vi "Get DQMH Main VI QD.vi"(8 "error in (no error)":errorcluster, 11 "Library Ref in":refnum<vi>) -> (0 "error out":errorcluster, 2 "Main VI Ref":refnum<vi>, 3 "Library Ref out":refnum<vi>)   [LabVIEW 2017]
doc: "Returns the Main VI of the DQMH Module of the selected SubVI."
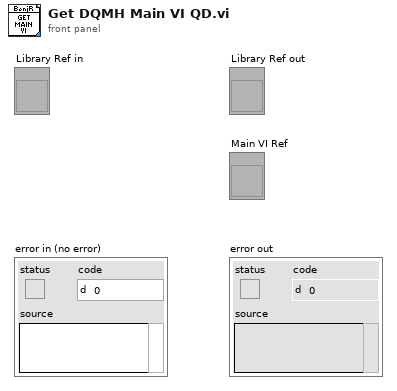
[diagram p1: front panel]
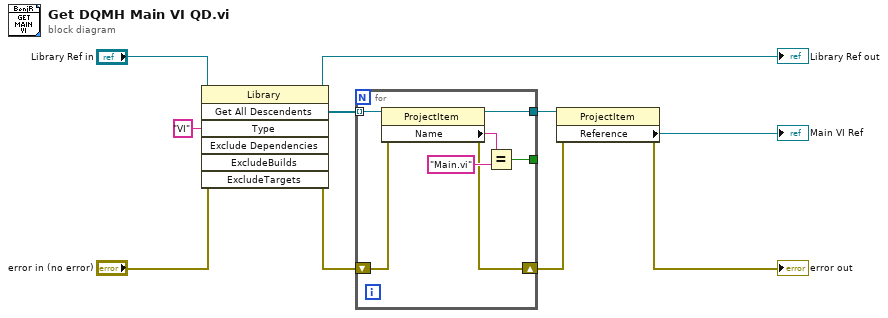
[diagram p0: block diagram]
diagram:
  n1 = invoke class="Library" method="Get All Descendents"(reference="Library Ref in", error in="error in (no error)", "Type"="VI") -> (reference out=→"Library Ref out":refnum<vi>, error out=w6:errorcluster, "All Descendents"=w3:refnum<vi>[])  [unwired: 4 in, 4 out]
  n2 = for {
    tunnel: w3 -> [w17] mode=indexing
    tunnel: [w14] -> _
    tunnel: [w13] -> w4
    shift-right: [w11] -> w7
    shift-left: w6 -> [w12]
    n3 = property class="ProjectItem"(reference=w17, error in=w12) -> (reference out=w13:refnum<vi>, error out=w11:errorcluster, "Name"=w16:string)
    n4 = Equal?(x=w16, y="Main.vi") -> (x = y?=w14:bool)
  }
  n5 = property class="ProjectItem"(reference=w4, error in=w7) -> (error out=→"error out":errorcluster, "Reference"=→"Main VI Ref":refnum<vi>)  [unwired: 1 out]
